vi "CurrentSource.vi"(0 "VISA resource name":refnum<visa-resource-name>, 1 "Timeout (10000 ms)":i32=10000 format="%#.6g", 5 "Number of Points (5)":u32=5, 7 "Compliance  Level (0.1)":dbl=0.1, 9 "Minimum Amplitude (1)":dbl=1.0, 11 "Maximum Amplitude (2)":dbl=2.0) -> (4 "B-fields":dbl[](array[numeric]))   [LabVIEW 2013]
doc: "Configures a sweep and takes voltage and current readings at each point."
uses:
  <instrlib>/Keithley 24XX/Public/Data/Read (Multiple Points).vi
  <instrlib>/Keithley 24XX/Keithley 24XX.lvlib
panel:
  out "Max Field /T":dbl
  out "Min Field /T\n /T":dbl
  in  "Output Mode":u16(ring)=1 items=["Fixed", "Sweep", "List"]
  in  "Serial Configuration":T1={"Baud Rate"=9600, "Parity"=0, "Data Bits"=8, "Stop Bits"=10, "Flow Control"=0} {"Flow Control" items=["None", "XON/XOFF", "RTS/CTS", "XON/XOFF & RTS/CTS", "DTR/DSR", "XON/XOFF & DTR/DSR"]; "Stop Bits" items=["1.0"=10, "1.5"=15, "2.0"=20]; "Data Bits" items=["7"=7, "8"=8]; "Parity" items=["None", "Odd", "Even", "Mark", "Space"]; "Baud Rate" items=["300"=300, "600"=600, "1200"=1200, "2400"=2400, "4800"=4800, "9600"=9600, "19200"=19200]}
  out "Waveform Graph":sgl[][](graph)
  # "(c) 2006 - 2015 National Instruments.  ALL RIGHTS RESERVED."
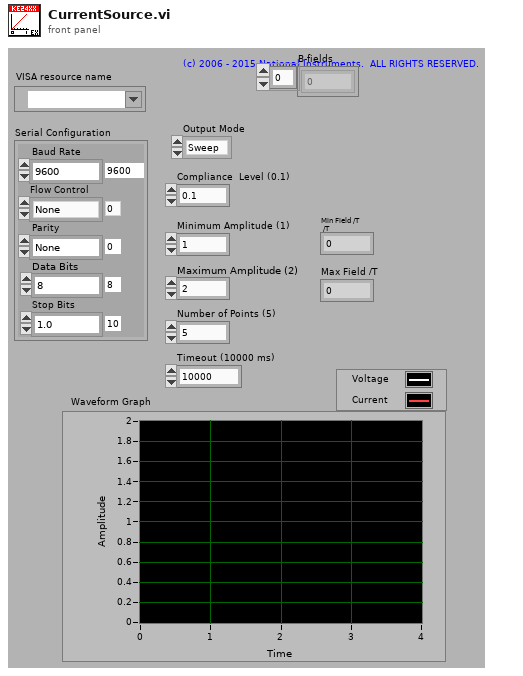
[diagram p1: front panel]
types:
  T1 = cluster{"Baud Rate":u32, "Parity":u16, "Data Bits":u16, "Stop Bits":u16, "Flow Control":u16}
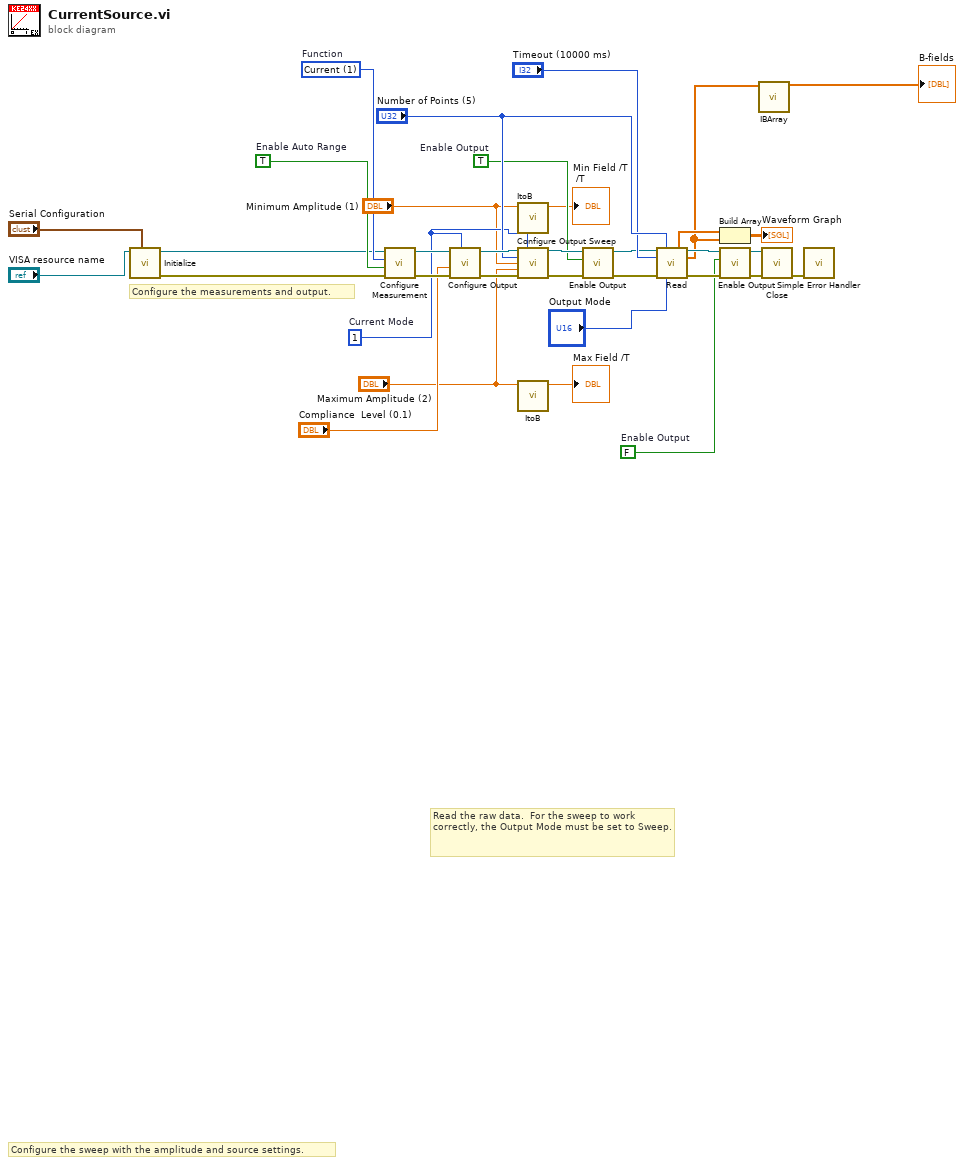
[diagram p0: block diagram]
diagram:
  w7 = u16 1  # Current Mode
  w10 = TRUE  # Enable Output
  w11 = TRUE  # Enable Auto Range
  w12 = u16 1 items=["Volts", "Current", "Resistance"]  # Function
  w18 = FALSE  # Enable Output
  # "Read the raw data.  For the sweep to work correctly, the Output Mode must be set to Sweep."
  # "Configure the sweep with the amplitude and source settings."
  # "Configure the measurements and output."
  n1 = call <instrlib>:"Initialize.vi"("Serial Configuration"="Serial Configuration", "VISA resource name"="VISA resource name") -> ("error out"=w8:errorcluster, "VISA resource name out"=w9:refnum<visa-resource-name>)  [unwired: 8 in]
  n2 = call <instrlib>:"Configure Measurement.vi"("error in (no error)"=w8, "Enable Auto Range (T:Enable)"=w11, "Function (0: Volts)"=w12, "VISA resource name"=w9) -> ("error out"=w33:errorcluster, "VISA resource name out"=w34:refnum<visa-resource-name>)  [unwired: 6 in]
  n3 = call <instrlib>:"Configure Output.vi"("Source Mode  (0: Voltage)"=w7, "error in (no error)"=w33, "Compliance  Level (0.1)"="Compliance  Level (0.1)", "VISA resource name"=w34) -> ("error out"=w32:errorcluster, "VISA resource name out"=w31:refnum<visa-resource-name>)  [unwired: 6 in]
  n4 = call "ItoB.vi"("Current"="Minimum Amplitude (1)") -> ("Field"=→"Min Field /T\n /T":dbl)  [unwired: 10 in]
  n5 = call <instrlib>:"Configure Output Sweep.vi"("VISA resource name"=w31, "Source Mode  (0: Voltage)"=w7, "Number of Points (5)"="Number of Points (5)", "Minimum Amplitude (1)"="Minimum Amplitude (1)", "Maximum Amplitude (2)"="Maximum Amplitude (2)", "error in (no error)"=w32) -> ("VISA resource name out"=w15:refnum<visa-resource-name>, "error out"=w14:errorcluster)  [unwired: 8 in]
  n6 = call "ItoB.vi"("Current"="Maximum Amplitude (2)") -> ("Field"=→"Max Field /T":dbl)  [unwired: 10 in]
  n7 = call <instrlib>:"Enable Output.vi"("error in (no error)"=w14, "Enable Output (T: Enable)"=w10, "VISA resource name"=w15) -> ("error out"=w17:errorcluster, "VISA resource name out"=w16:refnum<visa-resource-name>)  [unwired: 7 in]
  n8 = call-poly <instrlib>:"Read.vi"("VISA resource name"=w16, "Sample Count (1)"="Number of Points (5)", "Timeout (10000 ms)"="Timeout (10000 ms)", "error in (no error)"=w17, "Output Mode (0: Fixed)"="Output Mode") -> ("Voltage"=w28:sgl[], "VISA resource name out"=w19:refnum<visa-resource-name>, "Current"=w2:sgl[], "error out"=w20:errorcluster)  [unwired: 4 in, 3 out]
  n9 = Build Array(w28, w2) -> (→"Waveform Graph":sgl[][])
  n10 = call <instrlib>:"Enable Output.vi"("error in (no error)"=w20, "Enable Output (T: Enable)"=w18, "VISA resource name"=w19) -> ("error out"=w21:errorcluster, "VISA resource name out"=w22:refnum<visa-resource-name>)  [unwired: 7 in]
  n11 = call "IBArray.vi"("Current"=w2) -> ("Array"=→"B-fields":dbl[])  [unwired: 10 in]
  n12 = call <instrlib>:"Close.vi"("error in (no error)"=w21, "VISA resource name"=w22) -> ("error out"=w23:errorcluster)  [unwired: 9 in]
  n13 = call <vilib>:"Simple Error Handler.vi"("error in (no error)"=w23) -> ()  [unwired: 4 in, 5 out]
